vi "AxisWriteConf.vi"(6 "AditionalConfig":T1 {"UnitsControl" items=["mm", "°"]}, 8 "error in":errorcluster, 9 "AxisConfigurationIn":T2={"AxisHomeType"=1, "AxisBacklash"=0.0, "AxisGain"=1.0, "AxisOffset"=0.0, "AxisUnit"=1, "ReqConfRead"=FALSE, "ReqConfWrite"=FALSE, "AxisName"="", "AxisAccDecc"=0.0, "AxisHomeVel"=0.0} {"AxisUnit" items=["mm", "°"]; "AxisHomeType" items=["no homing"=0, "forward limit switch"=1, "backward limit switch"=2, "forward reference"=4, "backward reference"=8]}, 11 "Modbus master":refnum<class "Modbus Master.lvclass">) -> (0 "error out":errorcluster, 1 "AxisConfigurationOut":T2={"AxisHomeType"=1, "AxisBacklash"=0.0, "AxisGain"=1.0, "AxisOffset"=0.0, "AxisUnit"=1, "ReqConfRead"=FALSE, "ReqConfWrite"=FALSE, "AxisName"="", "AxisAccDecc"=0.0, "AxisHomeVel"=0.0} {"AxisUnit" items=["mm", "°"]; "AxisHomeType" items=["no homing"=0, "forward limit switch"=1, "backward limit switch"=2, "forward reference"=4, "backward reference"=8]})   [LabVIEW 2020, in "SMCD14_lib.lvlib"]
uses:
  SMCD14_lib.lvlib
  <vilib>/Modbus/master/Modbus Master.lvclass
  AxisConfiguration_typedef.ctl
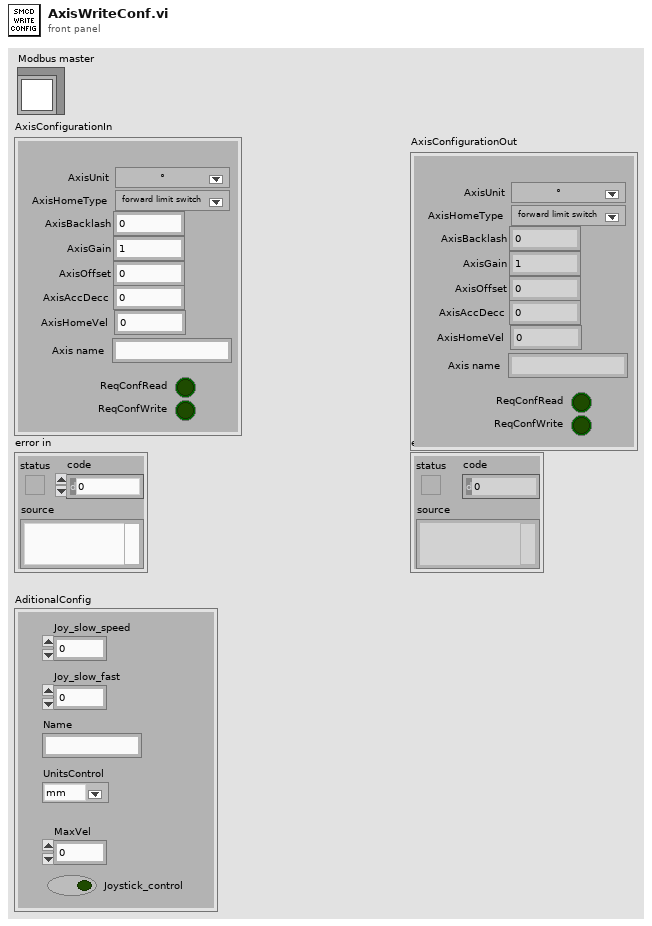
[diagram p1: front panel]
types:
  T1 = cluster{"Joy_slow_speed":sgl, "Joy_slow_fast":sgl, "Name":string, "UnitsControl":u16, "MaxVel":sgl, "Joystick_control":bool}
  T2 = typedef "SMCD14_lib.lvlib/AxisConfiguration_typedef.ctl" = cluster{"AxisHomeType":u16, "AxisBacklash":dbl, "AxisGain":dbl, "AxisOffset":dbl, "AxisUnit":u16, "ReqConfRead":bool, "ReqConfWrite":bool, "AxisName":string, "AxisAccDecc":dbl, "AxisHomeVel":dbl}
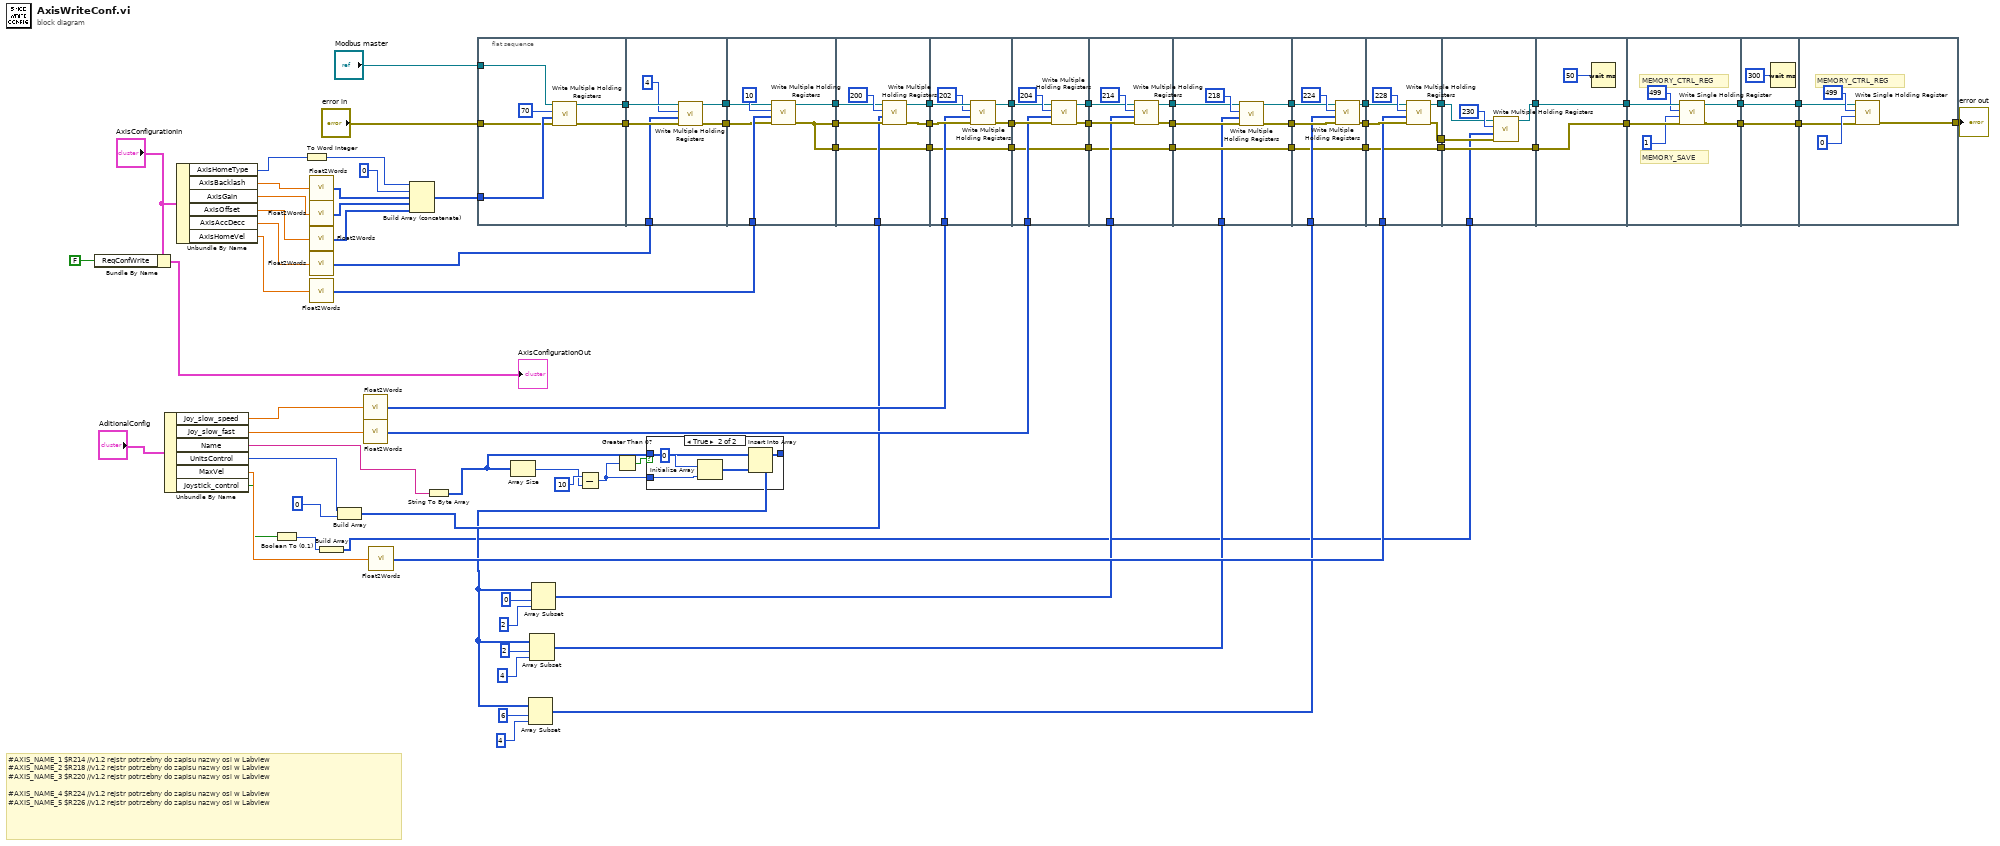
[diagram p0: block diagram]
diagram:
  # "#AXIS_NAME_1 $R214 //v1.2 rejstr potrzebny do zapisu nazwy osi w Labview\n#AXIS_NAME_2 $R218 //v1.2 rejstr potrzebny do zapisu nazwy osi w Labview\n#AXIS_NAME_3 $R220 //v1.2 rejstr potrzebny do zapisu nazwy osi w Labview\n\n#AXIS_NAME_4 $R224 //v1.2 rejstr potrzebny do zapisu nazwy osi w Labview\n#AXIS_NAME_5 $R226 //v1.2 rejstr potrzebny do zapisu nazwy osi w Labview"
  n1 = Bundle By Name(cluster="AxisConfigurationIn", "ReqConfWrite"=FALSE) -> (→"AxisConfigurationOut":T2)
  n2 = Unbundle By Name("AditionalConfig") -> ("Joy_slow_speed"=w54:sgl, "Joy_slow_fast"=w53:sgl, "Name"=w12:string, "UnitsControl"=w38:u16, "MaxVel"=w52:sgl, "Joystick_control"=w8:bool)
  n3 = Unbundle By Name("AxisConfigurationIn") -> ("AxisHomeType"=w82:u16, "AxisBacklash"=w80:dbl, "AxisGain"=w79:dbl, "AxisOffset"=w78:dbl, "AxisAccDecc"=w70:dbl, "AxisHomeVel"=w60:dbl)
  n4 = Boolean To (0,1)(Boolean=w8) -> (0, 1=w2:i16)
  n5 = To Word Integer(number=w82) -> (16bit integer=w81:i16)
  n6 = call "Float2Words.vi"("value"=w80) -> ("output"=w77:u16[])  [unwired: 4 in]
  n7 = call "Float2Words.vi"("value"=w79) -> ("output"=w76:u16[])  [unwired: 4 in]
  n8 = call "Float2Words.vi"("value"=w78) -> ("output"=w75:u16[])  [unwired: 4 in]
  n9 = call "Float2Words.vi"("value"=w70) -> ("output"=w59:u16[])  [unwired: 4 in]
  n10 = call "Float2Words.vi"("value"=w60) -> ("output"=w56:u16[])  [unwired: 4 in]
  n11 = Build Array(w2) -> (w1:i16[])
  n12 = Build Array(w38, u16 0 ("element")) -> (w36:u16[])
  n13 = call "Float2Words.vi"("value"=w54) -> ("output"=w51:u16[])  [unwired: 4 in]
  n14 = call "Float2Words.vi"("value"=w53) -> ("output"=w48:u16[])  [unwired: 4 in]
  n15 = call "Float2Words.vi"("value"=w52) -> ("output"=w43:u16[])  [unwired: 4 in]
  n16 = Build Array (concatenate)(w81, u16 0 ("element"), w77, w76, w75) -> (w84:u16[])
  n17 = String To Byte Array(string=w12) -> (unsigned byte array=w11:u8[])
  n18 = flat-sequence {
    tunnel: "Modbus master" -> [w91]
    tunnel: w84 -> [w89]
    tunnel: "error in" -> [w88]
    tunnel: [w87] -> w69
    tunnel: [w86] -> w68
    tunnel: w69 -> [w96]
    tunnel: w68 -> [w97]
    tunnel: w59 -> [w94]
    tunnel: [w93] -> w58
    tunnel: [w92] -> w57
    tunnel: w58 -> [w101]
    tunnel: [w100] -> w42
    tunnel: w57 -> [w99]
    tunnel: [w98] -> w40
    tunnel: w56 -> [w102]
    tunnel: [w98] -> w31
    tunnel: w42 -> [w109]
    tunnel: [w107] -> w41
    tunnel: w40 -> [w108]
    tunnel: [w106] -> w39
    tunnel: w36 -> [w105]
    tunnel: [w104] -> w32
    tunnel: w31 -> [w104]
    tunnel: w41 -> [w117]
    tunnel: [w115] -> w50
    tunnel: w39 -> [w116]
    tunnel: [w114] -> w49
    tunnel: w51 -> [w112]
    tunnel: [w111] -> w33
    tunnel: w32 -> [w111]
    tunnel: w50 -> [w123]
    tunnel: [w121] -> w47
    tunnel: w49 -> [w122]
    tunnel: [w120] -> w46
    tunnel: w48 -> [w119]
    tunnel: [w118] -> w34
    tunnel: w33 -> [w118]
    tunnel: w47 -> [w130]
    tunnel: [w128] -> w23
    tunnel: w46 -> [w129]
    tunnel: [w127] -> w21
    tunnel: w25 -> [w126]
    tunnel: [w125] -> w19
    tunnel: w34 -> [w125]
    tunnel: w23 -> [w136]
    tunnel: [w134] -> w22
    tunnel: w21 -> [w135]
    tunnel: [w133] -> w20
    tunnel: w19 -> [w138]
    tunnel: [w138] -> w18
    tunnel: w17 -> [w132]
    tunnel: w22 -> [w144]
    tunnel: [w142] -> w45
    tunnel: w20 -> [w143]
    tunnel: [w141] -> w44
    tunnel: w24 -> [w140]
    tunnel: [w139] -> w35
    tunnel: w18 -> [w139]
    tunnel: w45 -> [w151]
    tunnel: [w149] -> w7
    tunnel: w44 -> [w150]
    tunnel: w43 -> [w148]
    tunnel: [w147] -> w5
    tunnel: w35 -> [w147]
    tunnel: [w146] -> w3
    tunnel: w7 -> [w156]
    tunnel: [w155] -> w6
    tunnel: w5 -> [w158]
    tunnel: [w158] -> w4
    tunnel: w3 -> [w154]
    tunnel: w1 -> [w153]
    tunnel: w6 -> [w160]
    tunnel: [w160] -> w67
    tunnel: [w159] -> w66
    tunnel: w4 -> [w159]
    tunnel: w67 -> [w167]
    tunnel: w66 -> [w166]
    tunnel: [w163] -> w64
    tunnel: [w162] -> w62
    tunnel: [w169] -> w65
    tunnel: w64 -> [w169]
    tunnel: [w168] -> w63
    tunnel: w62 -> [w168]
    tunnel: w65 -> [w173]
    tunnel: w63 -> [w172]
    tunnel: [w171] -> w61
    frame #0 {
      n19 = call-dynamic "Write Multiple Holding Registers.vi"("error in (no error)"=w88, "holding register values"=w89, "starting address"=u16 70, "Modbus master in"=w91) -> ("error out"=w87:errorcluster, "Modbus master out"=w86:refnum<class "Modbus Master.lvclass">)  [unwired: 6 in]
    }
    frame #1 {
      n20 = call-dynamic "Write Multiple Holding Registers.vi"("error in (no error)"=w96, "holding register values"=w94, "starting address"=u16 4, "Modbus master in"=w97) -> ("error out"=w92:errorcluster, "Modbus master out"=w93:refnum<class "Modbus Master.lvclass">)  [unwired: 6 in]
    }
    frame #2 {
      n21 = call-dynamic "Write Multiple Holding Registers.vi"("error in (no error)"=w99, "holding register values"=w102, "starting address"=u16 10, "Modbus master in"=w101) -> ("error out"=w98:errorcluster, "Modbus master out"=w100:refnum<class "Modbus Master.lvclass">)  [unwired: 6 in]
    }
    frame #3 {
      n22 = call-dynamic "Write Multiple Holding Registers.vi"("error in (no error)"=w108, "holding register values"=w105, "starting address"=u16 200, "Modbus master in"=w109) -> ("error out"=w106:errorcluster, "Modbus master out"=w107:refnum<class "Modbus Master.lvclass">)  [unwired: 6 in]
    }
    frame #4 {
      n23 = call-dynamic "Write Multiple Holding Registers.vi"("error in (no error)"=w116, "holding register values"=w112, "starting address"=u16 202, "Modbus master in"=w117) -> ("error out"=w114:errorcluster, "Modbus master out"=w115:refnum<class "Modbus Master.lvclass">)  [unwired: 6 in]
    }
    frame #5 {
      n24 = call-dynamic "Write Multiple Holding Registers.vi"("error in (no error)"=w122, "holding register values"=w119, "starting address"=u16 204, "Modbus master in"=w123) -> ("error out"=w120:errorcluster, "Modbus master out"=w121:refnum<class "Modbus Master.lvclass">)  [unwired: 6 in]
    }
    frame #6 {
      n25 = call-dynamic "Write Multiple Holding Registers.vi"("error in (no error)"=w129, "holding register values"=w126, "starting address"=u16 214, "Modbus master in"=w130) -> ("error out"=w127:errorcluster, "Modbus master out"=w128:refnum<class "Modbus Master.lvclass">)  [unwired: 6 in]
    }
    frame #7 {
      n26 = call-dynamic "Write Multiple Holding Registers.vi"("error in (no error)"=w135, "holding register values"=w132, "starting address"=u16 218, "Modbus master in"=w136) -> ("error out"=w133:errorcluster, "Modbus master out"=w134:refnum<class "Modbus Master.lvclass">)  [unwired: 6 in]
    }
    frame #8 {
      n27 = call-dynamic "Write Multiple Holding Registers.vi"("error in (no error)"=w143, "holding register values"=w140, "starting address"=u16 224, "Modbus master in"=w144) -> ("error out"=w141:errorcluster, "Modbus master out"=w142:refnum<class "Modbus Master.lvclass">)  [unwired: 6 in]
    }
    frame #9 {
      n28 = call-dynamic "Write Multiple Holding Registers.vi"("error in (no error)"=w150, "holding register values"=w148, "starting address"=u16 228, "Modbus master in"=w151) -> ("error out"=w146:errorcluster, "Modbus master out"=w149:refnum<class "Modbus Master.lvclass">)  [unwired: 6 in]
    }
    frame #10 {
      n29 = call-dynamic "Write Multiple Holding Registers.vi"("error in (no error)"=w154, "holding register values"=w153, "starting address"=u16 230, "Modbus master in"=w156) -> ("Modbus master out"=w155:refnum<class "Modbus Master.lvclass">)  [unwired: 6 in, 1 out]
    }
    frame #11 {
      n30 = Wait (ms)(milliseconds to wait=u32 50) -> ()  [unwired: 1 out]
    }
    frame #12 {
      # "MEMORY_SAVE"
      # "MEMORY_CTRL_REG"
      n31 = call-dynamic "Write Single Holding Register.vi"("error in (no error)"=w166, "holding register value"=u16 1, "address"=u16 499, "Modbus master in"=w167) -> ("error out"=w162:errorcluster, "Modbus master out"=w163:refnum<class "Modbus Master.lvclass">)  [unwired: 6 in]
    }
    frame #13 {
      n32 = Wait (ms)(milliseconds to wait=u32 300) -> ()  [unwired: 1 out]
    }
    frame #14 {
      # "MEMORY_CTRL_REG"
      n33 = call-dynamic "Write Single Holding Register.vi"("error in (no error)"=w172, "holding register value"=u16 0, "address"=u16 499, "Modbus master in"=w173) -> ("error out"=w171:errorcluster)  [unwired: 6 in, 1 out]
    }
  }
  n34 = Array Size(array=w11) -> (size(s)=w15:i32)
  n35 = Subtract(x=10 ("y"), y=w15) -> (x-y=w9:i32)
  n36 = Greater Than 0?(x=w9) -> (x > 0?=w10:bool)
  n37 = case shown="True" w10 {
    tunnel: w9 -> [_ w181]
    tunnel: [w176 w178] -> w14
    tunnel: w11 -> [w176 w177]
    frame False {
    }
    frame True {
      n38 = Initialize Array(u16 0 ("element"), w181) -> (w179:u16[])
      n39 = Insert Into Array(array=w177, new element=w179) -> (w178:u8[])  [unwired: 1 in]
    }
  }
  n40 = Array Subset(array=w14, index=6, length=4) -> (w24:u8[])
  n41 = Array Subset(array=w14, index=2, length=4) -> (w17:u8[])
  n42 = Array Subset(array=w14, index=0, length=2) -> (w25:u8[])
  "error out" <- w61
